vi "USB Multiplexor Controller_v2.vi"(10 "Pixel number on\nsample holder":u32 caption="Pixel number on sample holder", 11 "Sample holder number":i64) -> ()   [LabVIEW 2011]
uses:
  <vilib>/ULx/Create Channel.llb/ULx Create Channel (DO-Digital Output).vi
  <vilib>/ULx/Write.llb/ULx Write (Digital U32 1Chan 1Samp).vi
panel:
  in  "Port":refnum<k21>="Dev0/AuxPort"
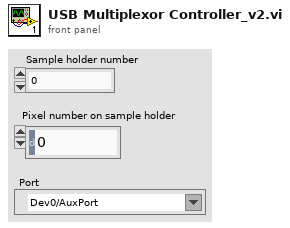
[diagram p1: front panel]
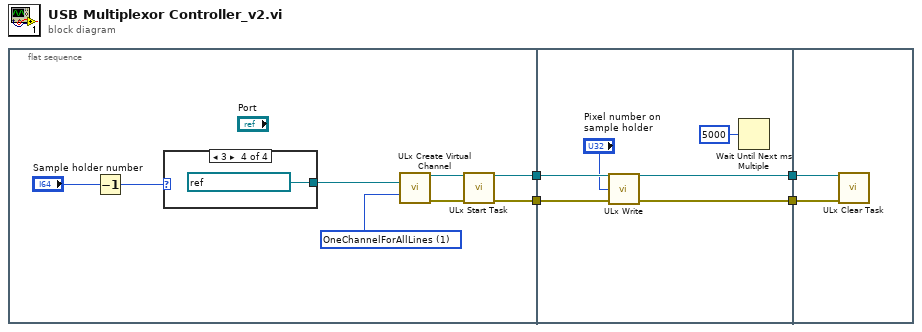
[diagram p0: block diagram]
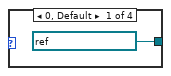
[diagram p2: hidden frame]
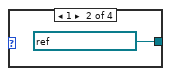
[diagram p3: hidden frame]
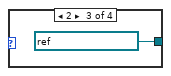
[diagram p4: hidden frame]
diagram:
  n1 = flat-sequence {
    tunnel: [w5] -> w4
    tunnel: [w6] -> w3
    tunnel: w4 -> [w22]
    tunnel: w3 -> [w20]
    tunnel: [w21] -> w2
    tunnel: [w19] -> w1
    tunnel: w2 -> [w23]
    tunnel: w1 -> [w24]
    frame #0 {
      w9 = 1 items=["OneChannelForEachLine", "OneChannelForAllLines"] ("line grouping")
      n2 = Decrement(x="Sample holder number") -> (x-1=w11:i64)
      n3 = case shown="3" w11 {
        tunnel: [refnum<k21> "Dev0/1stPortA" ("Port 2") refnum<k21> "Dev0/1stPortB" ("Port 2") refnum<k21> "Dev0/1stPortA" ("Port 2") refnum<k21> "Dev0/1stPortB" ("Port 2")] -> w12
        frame 0, Default {
        }
        frame 1 {
        }
        frame 2 {
        }
        frame 3 {
        }
      }
      n4 = call-poly <vilib>:"ULx Create Virtual Channel.vi"("lines"=w12, "line grouping"=w9) -> ("task out"=w7:refnum<k24>, "error out"=w8:errorcluster)  [unwired: 12 in]
      n5 = call <vilib>:"ULx Start Task.vi"("task in"=w7, "error in"=w8) -> ("task out"=w6:refnum<k24>, "error out"=w5:errorcluster)  [unwired: 12 in]
    }
    frame #1 {
      n6 = call-poly <vilib>:"ULx Write.vi"("task in"=w20, "data"="Pixel number on\nsample holder", "error in"=w22) -> ("task out"=w19:refnum<k24>, "error out"=w21:errorcluster)  [unwired: 10 in, 1 out]
      n7 = Wait Until Next ms Multiple(millisecond multiple=u32 5000 ("milliseconds to wait")) -> ()  [unwired: 1 out]
    }
    frame #2 {
      n8 = call <vilib>:"ULx Clear Task.vi"("task in"=w24, "error in"=w23) -> ()  [unwired: 13 in, 1 out]
    }
  }
